vi "JKI Rest Obj.vi"() -> (0 "REST Client_JKI":refnum<class "REST Client_JKI.lvclass">)   [LabVIEW 2018, in "REST Client.lvlib" / "REST Client_JKI.lvclass"]
uses:
  REST Client_JKI.lvclass
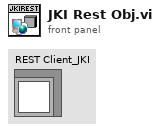
[diagram p1: front panel]
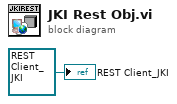
[diagram p0: block diagram]
diagram:
  "REST Client_JKI" <- refnum<class "REST Client_JKI.lvclass"> refnum ("REST Client.lvlib:REST Client_JKI.lvclass")
